vi "Error Display Window (Main).vi"(8 "Error In":errorcluster, 10 "Module Init Timestamp":timestamp, 11 "Error Details":T1) -> (0 "Error Out":errorcluster)   [LabVIEW 2016, in "Error Manager.lvlib" / "Error Display Window.lvclass"]
doc: "This is a user-facing window that displays to the user the error code, error message, and timestamp of a LabVIEW error that occured in the application.\n\n<B>Note</B>: Not necessarily every error that occurs in an application will be displayed by this dialogue. For example, if a while loop in an application starts producing the same error in a loop, and starts \"spamming\" the Error Manager module with dozens or hundreds of errors every second, if would be undesirable to popup this window once for every such error."
uses:
  Error Display Window.lvclass
  <vilib>/Utility/error.llb/DialogType.ctl
  Error Manager.lvlib
  Private VIs/Close Window Option (Enum).ctl
  Settings/Settings.lvclass
  Error Details (cluster).ctl
panel:
  out "Clipboard Confirmation Message":string
  out "Error Code":string
  in  "Copy Error Details To Clipboard":bool
  out "Timestamp":string
  out "Error Message":string
  in  "Sizing Tool":bool
  in  "OK Button":bool
  out "EHL iteration":i32
  out "Pre-loop Init":errorcluster
  # "User-facing region."
  # "Error"
  # "Non-user-facing region. Developer-facing only."
  # "Input\nInputs to the VI"
  # "Development\ncontrols/indicators useful for development and testing, but which are not outputs of the VI"
  # "Output\nOutputs of the VI"
  # "The Error Out indicator is larger than usual in order to be able to view the full error message without having to scroll."
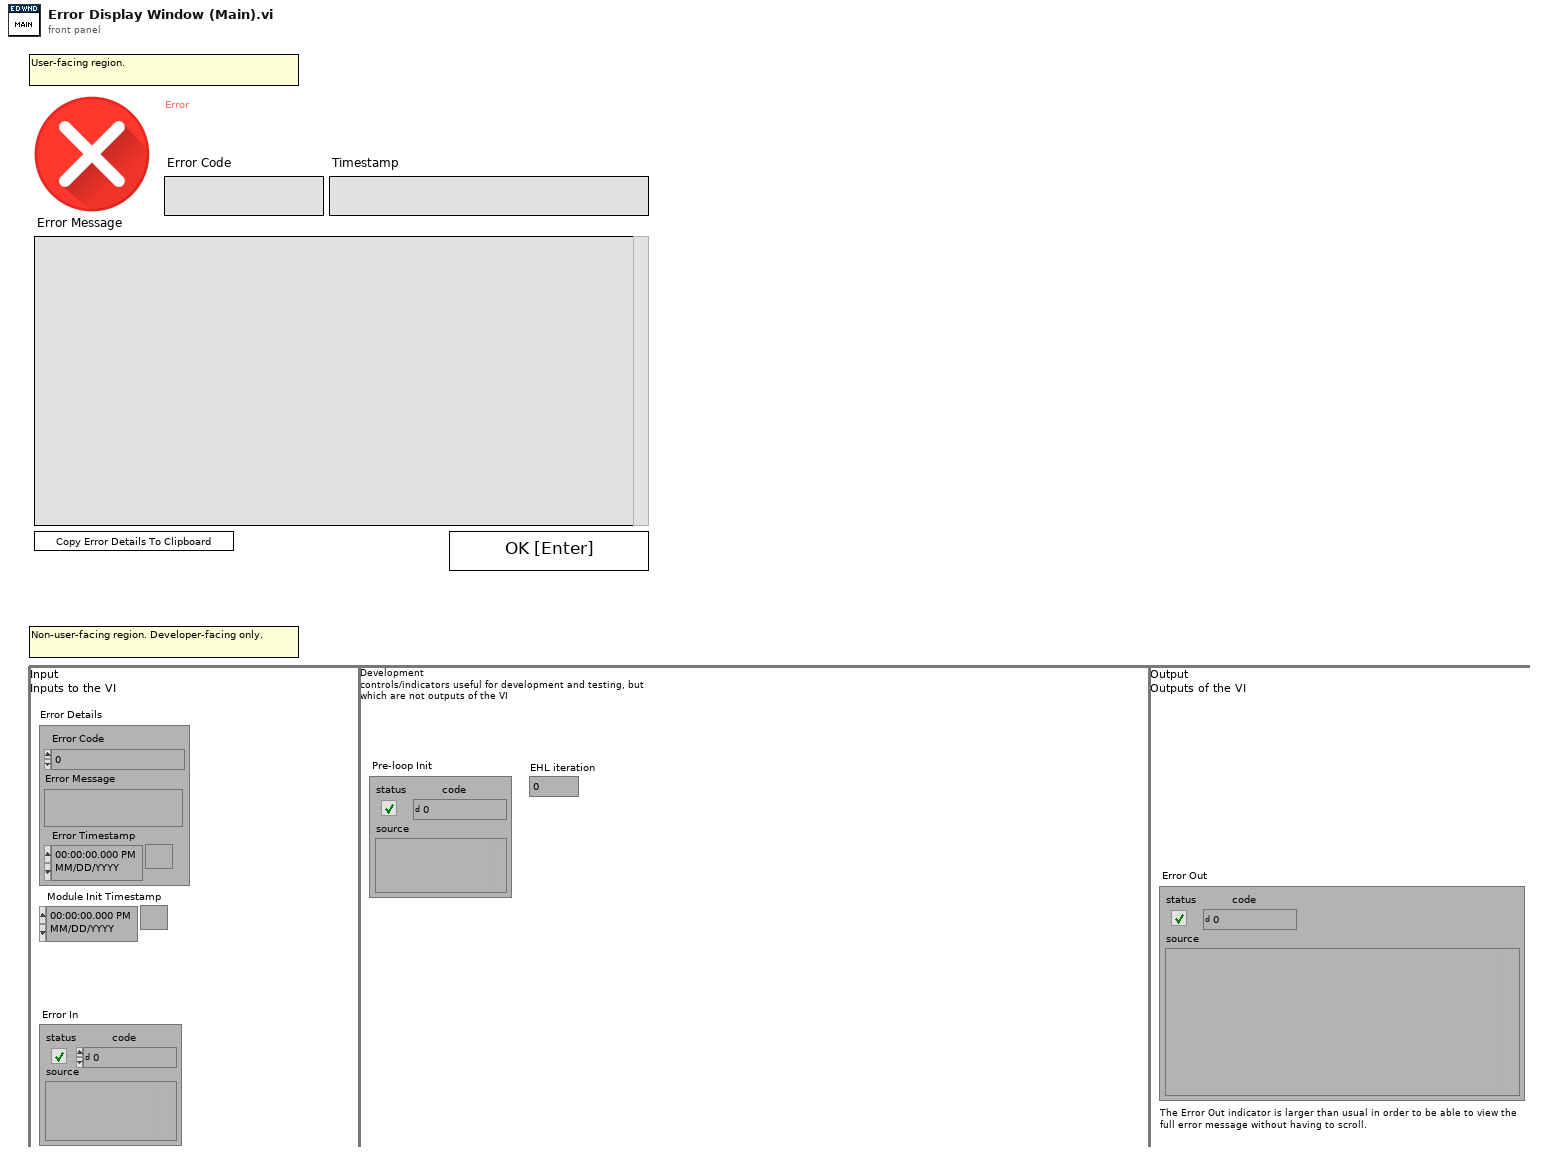
[diagram p1: front panel]
types:
  T1 = typedef "Error Manager.lvlib/Error Display Window.lvclass/Error Details (cluster).ctl" = cluster{"Error Code":i32, "Error Message":string, "Error Timestamp":timestamp}
  T2 = typedef "Error Manager.lvlib/Close Window Option (Enum).ctl" = enum16{"In dev env, don't close", "In dev env, don't close if top-level caller", "Close Always"}
  T3 = typedef "Error Manager.lvlib/Settings.lvclass/Window_Behaviour (enum).ctl" = enum16{"Default", "Floating", "Modal"}
  T4 = typedef "DialogType.ctl" = u16
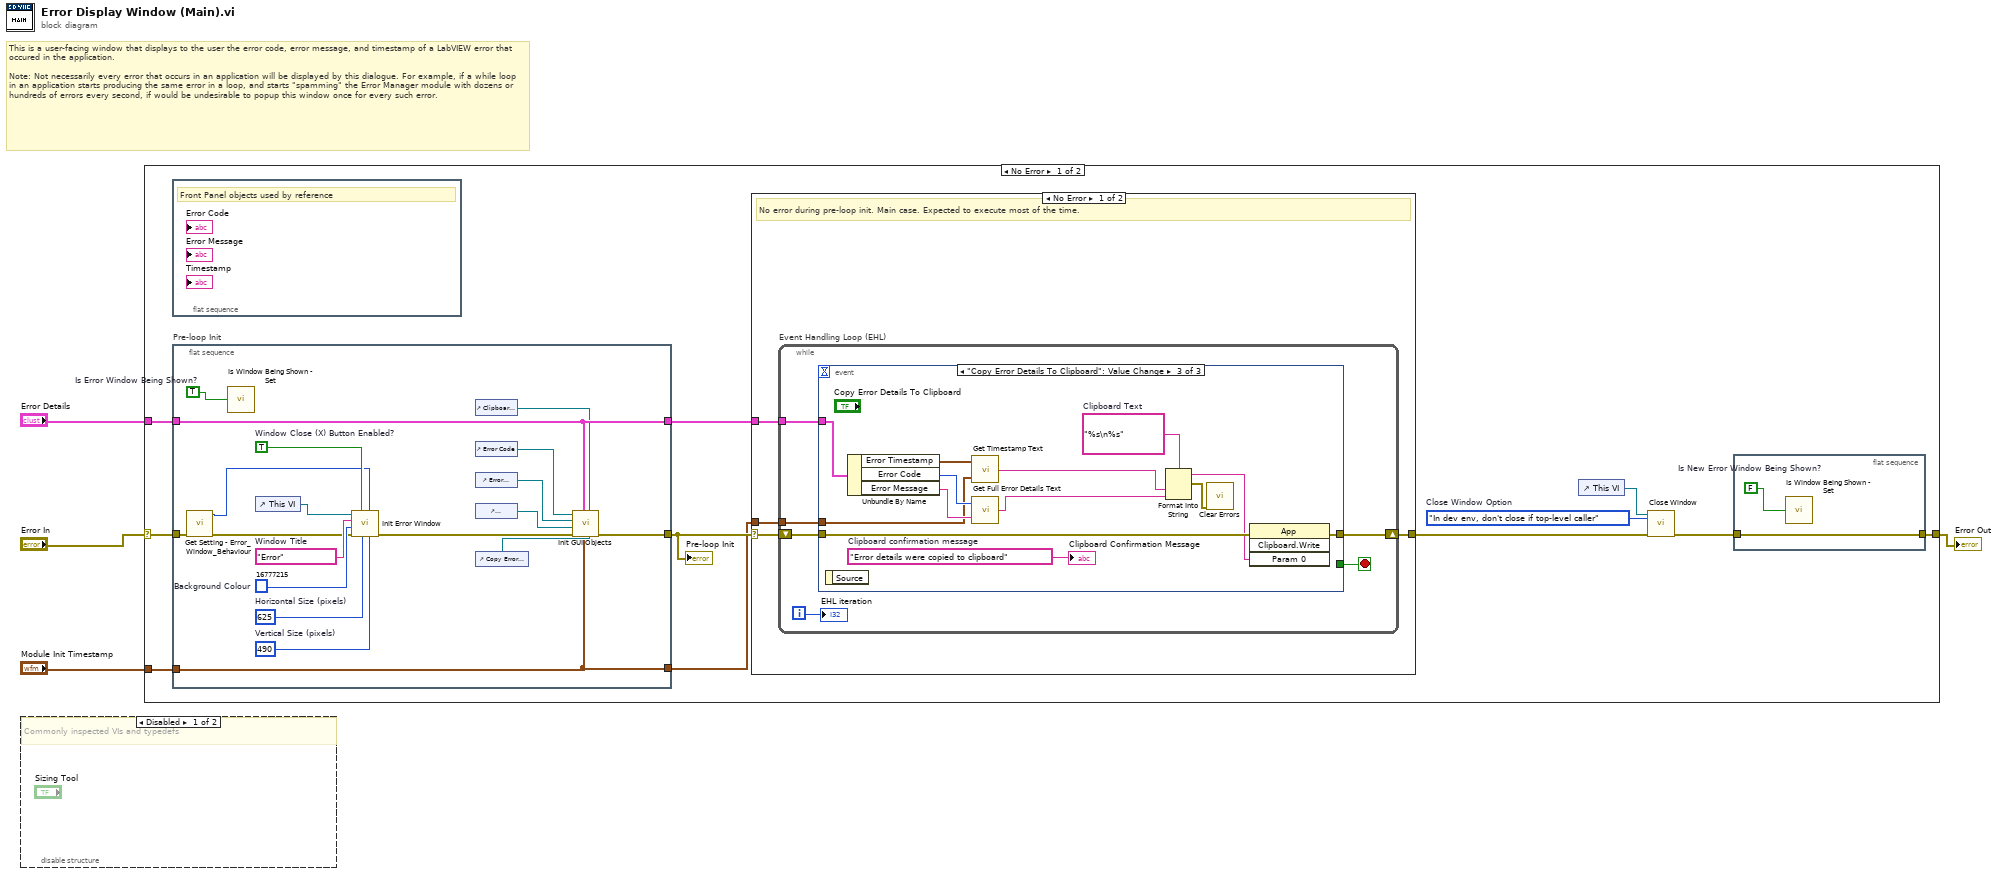
[diagram p0: block diagram]
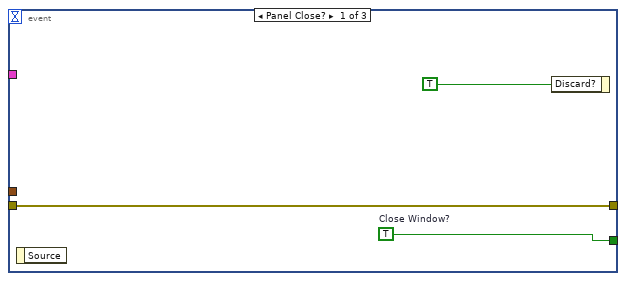
[diagram p2: hidden frame]
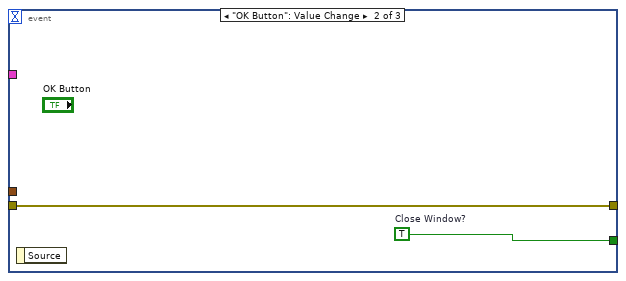
[diagram p3: hidden frame]
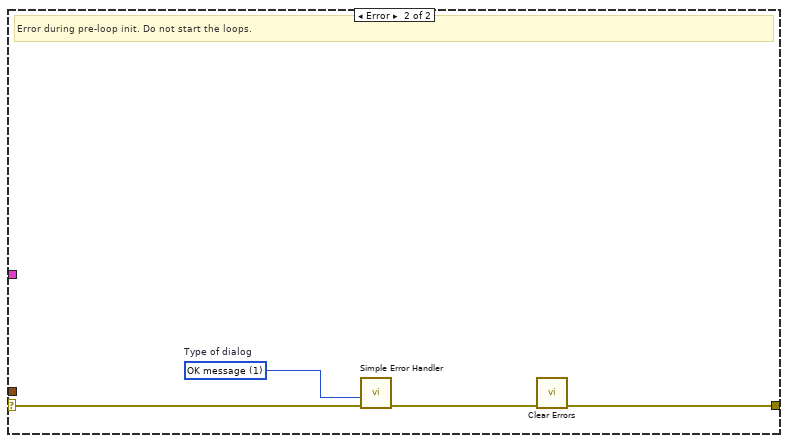
[diagram p4: hidden frame]
diagram:
  # "This is a user-facing window that displays to the user the error code, error message, and timestamp of a LabVIEW error that occured in the application.\n\nNote: Not necessarily every error that occurs in an application will be displayed by this dialogue. For example, if a while loop in an application starts producing the same error in a loop, and starts \"spamming\" the Error Manager module with dozens or hundreds of errors every second, if would be undesirable to popup this window once for every such error."
  n1 = disable-structure shown="Disabled" {
    frame Disabled {
      # "Commonly inspected VIs and typedefs"
    }
    frame Enabled {
    }
  }
  n2 = case shown="No Error" "Error In" {
    selector: "Error In" -> [w14 w69]
    tunnel: [w13 w69] -> w4
    tunnel: "Error Details" -> [w12 _]
    tunnel: "Module Init Timestamp" -> [w7 _]
    frame No Error {
      w8 = Close_Window_Option_(Enum)."In dev env, don't close if top-level caller"  # Close Window Option
      n3 = flat-sequence {
        frame #0 {
          # "Front Panel objects used by reference"
        }
      }
      n4 = flat-sequence "Pre-loop Init" {
        tunnel: [w29] -> w15
        tunnel: w14 -> [w30]
        tunnel: w12 -> [w20]
        tunnel: w7 -> [w19]
        tunnel: [w20] -> w6
        tunnel: [w19] -> w5
        frame #0 {
          w26 = TRUE  # Window Close (X) Button Enabled?
          w27 = u32 16777215  # Background Colour
          w33 = i16 490  # Vertical Size (pixels)
          w32 = i16 625  # Horizontal Size (pixels)
          w31 = "Error"  # Window Title
          w36 = TRUE  # Is Error Window Being Shown?
          n5 = call "Get Setting - Error_Window_Behaviour.vi"("Error In"=w30) -> ("Error Out"=w25:errorcluster, "Error_Window_Behaviour"=w24:T3)  [unwired: 9 in]
          n6 = call "Is Window Being Shown - Set.vi"("Is Window Being Shown?"=w36) -> ()
          n7 = control-ref of="This VI"() -> (w34:refnum<vi>)
          n8 = call "Init Error Window.vi"("Window Vertical Size (pixels)"=w33, "Window Behaviour"=w24, "Window Horizontal Size (pixels)"=w32, "Window Close (X) Button Enabled? (Default = True)"=w26, "error in"=w25, "Background Colour (Default = 255,255,255)"=w27, "Window Title"=w31, "VI Refnum"=w34) -> ("error out"=w28:errorcluster)  [unwired: 3 in]
          n9 = control-ref of="Clipboard Confirmation Message"() -> (w18:refnum<vi>)
          n10 = control-ref of="Error Code"() -> (w23:refnum<vi>)
          n11 = control-ref of="Error Message"() -> (w35:refnum<vi>)
          n12 = control-ref of="Timestamp"() -> (w22:refnum<vi>)
          n13 = control-ref of="Copy Error Details To Clipboard"() -> (w21:refnum<vi>)
          n14 = call "Init GUI Objects.vi"("Copy Error Details To Clipboard"=w21, "Clipboard Confirmation Message"=w18, "Module Init Timestamp"=w19, "Error Details"=w20, "error in"=w28, "Timestamp"=w22, "Error Message"=w35, "Error Code"=w23) -> ("error out"=w29:errorcluster)  [unwired: 3 in]
        }
      }
      n15 = case shown="No Error" w15 {
        selector: w15 -> [w39 w68]
        tunnel: [w40 w66] -> w10
        tunnel: w6 -> [w38 _]
        tunnel: w5 -> [w37 _]
        frame No Error {
          # "No error during pre-loop init. Main case. Expected to execute most of the time."
          n16 = while "Event Handling Loop (EHL)" {
            shift-right: [w44] -> w40
            shift-left: w39 -> [w46]
            tunnel: w38 -> [w42]
            tunnel: w37 -> [w41]
            i -> [w43]
            stop <- w45 stop-if-true
            n17 = event shown="[2] \"Copy Error Details To Clipboard\": Value Change" {
              selector: _ -> [_ _ _]
              dyn-events: _ -> [_ _ _]
              timeout: _ -> [_ _ _]
              tunnel: w46 -> [w48 w51 w64]
              tunnel: [w47 w50 _] -> w45
              tunnel: [w48 w51 w63] -> w44
              tunnel: w42 -> [_ _ w57]
              tunnel: w41 -> [_ _ w53]
              event Panel Close? {
                w47 = TRUE  # Close Window?
                n18 = event-data() -> ()  [unwired: 1 in, 1 out]
                n19 = event-data("Discard?"=TRUE) -> ()  [unwired: 1 in, 1 out]
              }
              event "OK Button": Value Change {
                w50 = TRUE  # Close Window?
                n20 = event-data() -> ()  [unwired: 1 in, 1 out]
              }
              event "Copy Error Details To Clipboard": Value Change {
                w52 = "Error details were copied to clipboard"  # Clipboard confirmation message
                w61 = "%s\n%s"  # Clipboard Text
                n21 = event-data() -> ()  [unwired: 1 in, 1 out]
                n22 = Unbundle By Name(w57) -> ("Error Timestamp"=w54:timestamp, "Error Code"=w56:i32, "Error Message"=w55:string)
                n23 = call "Get Timestamp Text.vi"("Module Init Timestamp"=w53, "Error Timestamp"=w54) -> ("Timestamp String"=w59:string)
                n24 = call "Get Full Error Details Text.vi"("Error Message"=w55, "Error Code"=w56) -> ("Full Error Details Text"=w58:string)
                n25 = Format Into String(format string=w61, w59, w58) -> (resulting string=w60:string, error out=w62:errorcluster)  [unwired: 2 in]
                n26 = call <vilib>:"Clear Errors.vi"("error in (no error)"=w62) -> ()  [unwired: 5 in, 2 out]
                n27 = invoke class="App" method="Clipboard.Write"(error in=w64, "Param 0"=w60) -> (error out=w63:errorcluster)  [unwired: 2 in, 3 out]
                "Clipboard Confirmation Message" <- w52
              }
            }
            "EHL iteration" <- w43
          }
        }
        frame Error {
          w65 = T4 1 items=["no dialog", "OK message", "continue or stop message", "OK message + warnings", "continue/stop + warnings"]  # Type of dialog
          # "Error during pre-loop init. Do not start the loops."
          n28 = call <vilib>:"Simple Error Handler.vi"("type of dialog (OK msg:1)"=w65, "error in (no error)"=w68) -> ("error out"=w67:errorcluster)  [unwired: 3 in, 4 out]
          n29 = call <vilib>:"Clear Errors.vi"("error in (no error)"=w67) -> ("error out"=w66:errorcluster)  [unwired: 5 in, 1 out]
        }
      }
      n30 = control-ref of="This VI"() -> (w11:refnum<vi>)
      n31 = call "Close Window.vi"("error in"=w10, "Close Window Option (Default = \"In dev env, don't close if top-level caller\")"=w8, "VI Refnum"=w11) -> ("error out"=w9:errorcluster)  [unwired: 8 in]
      n32 = flat-sequence {
        tunnel: [w17] -> w13
        tunnel: w9 -> [w17]
        frame #0 {
          w16 = FALSE  # Is New Error Window Being Shown?
          n33 = call "Is Window Being Shown - Set.vi"("Is Window Being Shown?"=w16) -> ()
        }
      }
      "Pre-loop Init" <- w15
    }
    frame Error {
      # "Error upstream. Do nothing."
    }
  }
  "Error Out" <- w4
